vi "Convert Homography to Pose.vi"(6 "filter":T1, 9 "Scale to Inches":dbl[](array[numeric])=[-2.8, 1.0, 4.1], 10 "Inverse Camera Matrix":T3, 11 "tag info":T2={"tag ID"=0, "Center (pix)"={"X"=0.0, "Y"=0.0}, "homography matrix"=[], "score"=0.0, "Hamming Dist"=0, "corners (pix)"=[], "Tag Family"="36h11"}) -> (1 "Translation":dbl[](array[numeric]), 2 "angles SVD":cluster{"roll":dbl, "pitch":dbl, "yaw":dbl}, 3 "angles (deg)":cluster{"yaw":dbl, "pitch":dbl, "roll":dbl})   [LabVIEW 2025]
uses:
  <vilib>/Analysis/Matrix/Datatypes/RealMatrix.ctl
  filter Selector.ctl
  <vilib>/Analysis/baseanly.llb/Real A x B.vi
  <vilib>/Analysis/_algsub.llb/Real Vector Norm.vi
  <vilib>/Analysis/7linalg.llb/Real Transpose Matrix.vi
  <vilib>/Analysis/baseanly.llb/A x Vector.vi
  <vilib>/Analysis/Matrix/Numeric/Multiply/Multiply - R,RM.vi
  <vilib>/addons/control/pid/pid.llb/PID Control Input Filter (DBL Array).vi
  <vilib>/Analysis/NI_AALBase.lvlib
  <vilib>/Analysis/NI_AALPro.lvlib
  <vilib>/robotics/Kinematics/NI_Kinematics.lvlib
  <vilib>/Analysis/Matrix/NI_Matrix.lvlib
  <vilib>/Analysis/7linalg.llb/SVD Option.ctl
  <vilib>/Analysis/7linalg.llb/Real SVD Decomposition.vi
  <vilib>/addons/control/pid/NI_PID_pid.lvlib
  <vilib>/ptbypt/NI_PtbyPt.lvlib
panel:
  in  "median rank":i32=1
  out "raw translation":dbl[](array[numeric])
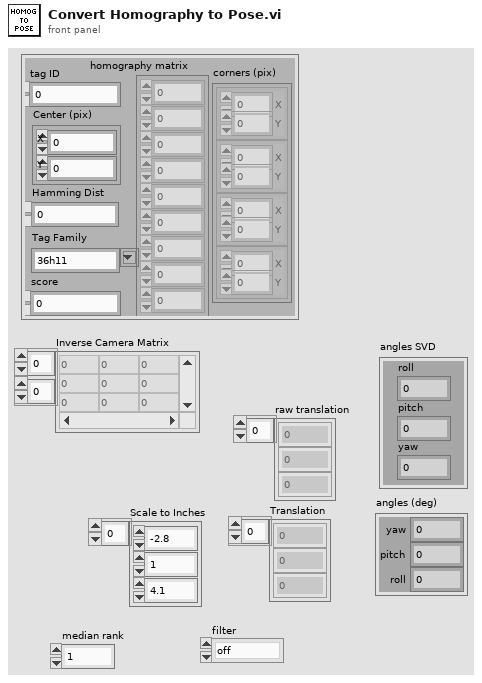
[diagram p1: front panel]
types:
  T1 = typedef "filter Selector.ctl" = enum16{"off", "2 pt avg", "low pass"}
  T2 = cluster{"tag ID":i32, "Center (pix)":cluster{"X":dbl, "Y":dbl}, "homography matrix":dbl[], "score":dbl, "Hamming Dist":i32, "corners (pix)":cluster{"X":dbl, "Y":dbl}[], "Tag Family":string}
  T3 = typedef "NI_Matrix.lvlib/RealMatrix.ctl" = dbl[][]
  T4 = typedef "NI_AALPro.lvlib/SVD Option.ctl" = u16
  T5 = cluster{"Filtered x":dbl, "Filtered x":dbl, "Filtered x":dbl}
  T6 = cluster{"output[0]":dbl, "output[1]":dbl, "output[2]":dbl}
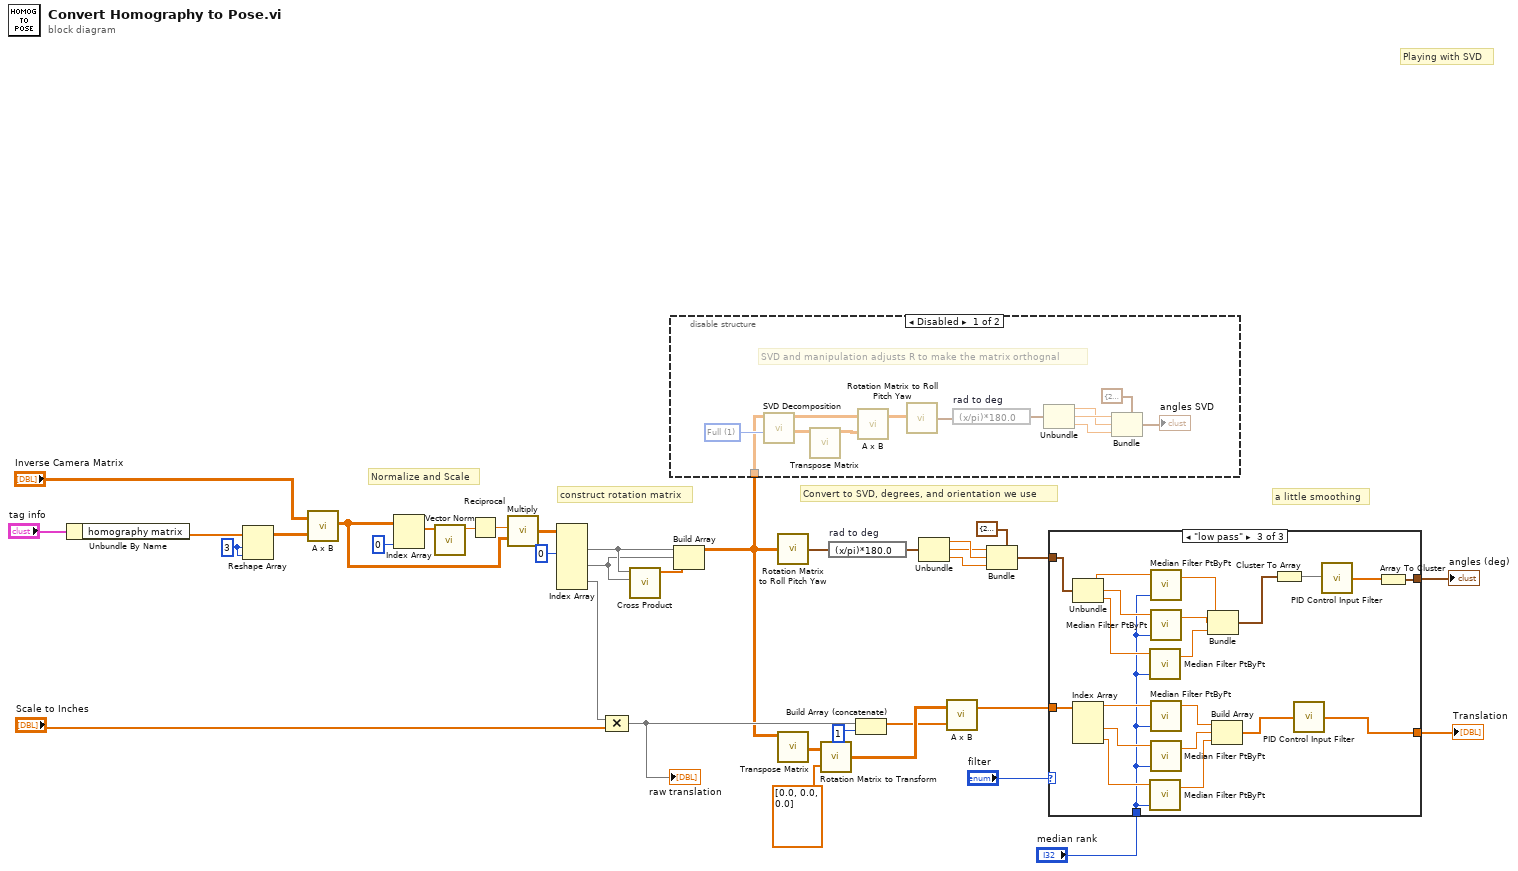
[diagram p0: block diagram]
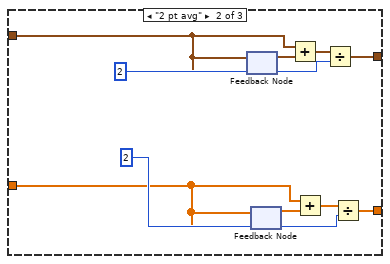
[diagram p3: hidden frame]
diagram:
  w36 = 3 ("dimension size")
  # "a little smoothing"
  # "Convert to SVD, degrees, and orientation we use"
  # "construct rotation matrix"
  # "Normalize and Scale"
  # "Playing with SVD"
  n1 = Unbundle By Name("tag info") -> ("homography matrix"=w4:dbl[])
  n2 = Reshape Array(w4, w36, w36) -> (w3:dbl[][])
  n3 = call-poly <vilib>:"A x B.vi"("B"=w3, "A"="Inverse Camera Matrix") -> ("A x B"=w30:T3)  [unwired: 1 out]
  n4 = Index Array(array=w30, index (col)=0 ("disabled index (col)")) -> (element=w32:dbl[])  [unwired: 1 in]
  n5 = call-poly <vilib>:"Vector Norm.vi"("Input Vector"=w32) -> ("norm"=w33:dbl)  [unwired: 9 in, 1 out]
  n6 = Reciprocal(x=w33) -> (1/x=w31:dbl)
  n7 = call-poly <vilib>:"Multiply.vi"("Real Matrix A"=w30, "Real Scalar c"=w31) -> ("c * A"=w28:T3)
  n8 = Index Array(array=w28, index (col) #1=0 ("disabled index (col)")) -> (element #1=w27:dbl[], element #2=w26:dbl[], element #3=w18:dbl[])  [unwired: 5 in]
  n9 = Compound Arithmetic op=MULTIPLY(w18, "Scale to Inches") -> (w15:dbl[])
  "raw translation" <- w15
  n10 = call <vilib>:"Cross Product.vi"("B Vector"=w26, "A Vector"=w27) -> ("Cross Product"=w25:dbl[])  [unwired: 8 in, 1 out]
  n11 = Build Array(w27, w26, w25) -> (w11:T3)
  n12 = disable-structure shown="Disabled" {
    disable-tunnel: w11 -> [w43 _]
    frame Disabled {
      w47 = T4 1 items=["Thin", "Full"] ("SVD option")
      # "SVD and manipulation adjusts R to make the matrix orthognal"
      n13 = call-poly <vilib>:"SVD Decomposition.vi"("SVD option"=w47, "A"=w43) -> ("Matrix V"=w45:T3, "Matrix U"=w49:T3)  [unwired: 5 in, 3 out]
      n14 = call-poly <vilib>:"Transpose Matrix.vi"("Input Matrix"=w45) -> ("Matrix Transpose"=w44:T3)  [unwired: 9 in, 1 out]
      n15 = call-poly <vilib>:"A x B.vi"("B"=w44, "A"=w49) -> ("A x B"=w46:T3)  [unwired: 1 out]
      n16 = call <vilib>:"Rotation Matrix to Roll Pitch Yaw.vi"("rotation matrix"=w46) -> ("angles"=w48:cluster{"roll":dbl, "pitch":dbl, "yaw":dbl})
      n17 = expression code="(x/pi)*180.0" "rad to deg"(w48) -> (w38:cluster{"roll":dbl, "pitch":dbl, "yaw":dbl})
      n18 = Unbundle(w38) -> ("roll"=w39:dbl, "pitch"=w42:dbl, "yaw"=w40:dbl)
      n19 = Bundle(cluster=cluster{"yaw":dbl, "pitch":dbl, "roll":dbl} {"yaw"=25.18811270112165, "pitch"=-30.885572547805758, "roll"=-2.4619221233355195} ("YPR (deg)"), "yaw"=w42, "pitch"=w39, "roll"=w40) -> (→"angles SVD":cluster{"yaw":dbl, "pitch":dbl, "roll":dbl})
    }
    frame Enabled {
    }
  }
  n20 = call <vilib>:"Rotation Matrix to Roll Pitch Yaw.vi"("rotation matrix"=w11) -> ("angles"=w17:cluster{"roll":dbl, "pitch":dbl, "yaw":dbl})
  n21 = call-poly <vilib>:"Transpose Matrix.vi"("Input Matrix"=w11) -> ("Matrix Transpose"=w10:T3)  [unwired: 9 in, 1 out]
  n22 = call <vilib>:"Rotation Matrix to Transform.vi"("translation vector"=dbl[] [0.0, 0.0, 0.0] ("subarray"), "rotation matrix"=w10) -> ("transform"=w16:T3)
  n23 = expression code="(x/pi)*180.0" "rad to deg"(w17) -> (w20:cluster{"roll":dbl, "pitch":dbl, "yaw":dbl})
  n24 = Build Array (concatenate)(w15, 1 ("dimension size")) -> (w12:dbl[])
  n25 = Unbundle(w20) -> ("roll"=w24:dbl, "pitch"=w21:dbl, "yaw"=w23:dbl)
  n26 = call-poly <vilib>:"A x B.vi"("Vector"=w12, "A"=w16) -> ("A x Vector"=w7:dbl[])  [unwired: 1 out]
  n27 = Bundle(cluster=cluster{"yaw":dbl, "pitch":dbl, "roll":dbl} {"yaw"=25.18811270112165, "pitch"=-30.885572547805758, "roll"=-2.4619221233355195} ("YPR (deg)"), "yaw"=w21, "pitch"=w24, "roll"=w23) -> (w9:cluster{"yaw":dbl, "pitch":dbl, "roll":dbl})
  n28 = case shown="\"low pass\"" "filter" {
    tunnel: w9 -> [w51 w55 w71]
    tunnel: [w51 w54 w79] -> w8
    tunnel: w7 -> [w50 w53 w70]
    tunnel: [w50 w52 w82] -> w6
    tunnel: "median rank" -> [_ _ w62]
    frame "off", Default {
    }
    frame "2 pt avg" {
      n29 = feedback #1(w55) -> (w60:cluster{"yaw":dbl, "pitch":dbl, "roll":dbl})
      n30 = feedback-in #1(w55) -> ()
      n31 = feedback #2(w53) -> (w61:dbl[])
      n32 = feedback-in #2(w53) -> ()
      n33 = Add(x=w55, y=w60) -> (x+y=w59:cluster{"yaw":dbl, "pitch":dbl, "roll":dbl})
      n34 = Add(x=w53, y=w61) -> (x+y=w58:dbl[])
      n35 = Divide(x=w59, y=2 ("disabled index (col)")) -> (x/y=w54:cluster{"yaw":dbl, "pitch":dbl, "roll":dbl})
      n36 = Divide(x=w58, y=2 ("disabled index (col)")) -> (x/y=w52:dbl[])
    }
    frame "low pass" {
      n37 = Unbundle(w71) -> ("yaw"=w78:dbl, "pitch"=w77:dbl, "roll"=w76:dbl)
      n38 = Index Array(array=w70) -> (element #1=w69:dbl, element #2=w68:dbl, element #3=w67:dbl)  [unwired: 3 in]
      n39 = call <vilib>:"Median Filter PtByPt.vi"("rank"=w62, "x"=w76) -> ("Filtered x"=w73:dbl)  [unwired: 2 in, 1 out]
      n40 = call <vilib>:"Median Filter PtByPt.vi"("rank"=w62, "x"=w67) -> ("Filtered x"=w64:dbl)  [unwired: 2 in, 1 out]
      n41 = call <vilib>:"Median Filter PtByPt.vi"("rank"=w62, "x"=w78) -> ("Filtered x"=w75:dbl)  [unwired: 2 in, 1 out]
      n42 = call <vilib>:"Median Filter PtByPt.vi"("rank"=w62, "x"=w77) -> ("Filtered x"=w74:dbl)  [unwired: 2 in, 1 out]
      n43 = call <vilib>:"Median Filter PtByPt.vi"("rank"=w62, "x"=w69) -> ("Filtered x"=w66:dbl)  [unwired: 2 in, 1 out]
      n44 = call <vilib>:"Median Filter PtByPt.vi"("rank"=w62, "x"=w68) -> ("Filtered x"=w65:dbl)  [unwired: 2 in, 1 out]
      n45 = Bundle("Filtered x"=w75, "Filtered x"=w74, "Filtered x"=w73) -> (w72:T5)  [unwired: 1 in]
      n46 = Build Array(w66, w65, w64) -> (w63:dbl[])
      n47 = Cluster To Array(cluster=w72) -> (array=w81:dbl[])
      n48 = call-poly <vilib>:"PID Control Input Filter.vi"("input"=w63) -> ("output"=w82:dbl[])  [unwired: 4 in]
      n49 = call-poly <vilib>:"PID Control Input Filter.vi"("input"=w81) -> ("output"=w80:dbl[])  [unwired: 4 in]
      n50 = Array To Cluster(array=w80) -> (cluster=w79:T6)
    }
  }
  "angles (deg)" <- w8
  "Translation" <- w6
